vi "THzTimeScan_830_VC_PSD_TA_170401.vi"(0 "input":T1={"Step Number"=0, "Step"=0.0, "Start Position"=0.0, "Time-out"=0, "Lockin Address"="", "Short term \nAverage#"=0, "ESP300 Axis"=0, "error in"={"status"=FALSE, "code"=0, "source"=""}, "Value"="", "Delay"=0.0, "Delay2"=0.0, "savepath"=path "", "Power meter"={"ConexPSD Reference"=refnum, "error out"={"status"=FALSE, "code"=0, "source"=""}, "Component ID"=1}}) -> (1 "loop stop":bool, 2 "x-axis":sgl[](array[numeric]), 3 "y-axis":dbl[](array[numeric]), 4 "ext. out":cluster{dbl[], dbl[], dbl[], dbl[], string[]})   [LabVIEW 2010]
uses:
  C:/Users/NBTP/Desktop/Tai Anh/1. Courses + Small Works/Graduation Project/LabVIEW/TDS LabVIEW/THz Time(ESP300&SR830&PSD&MCS) TA_170209/Dll/Newport.CONEXPSD.CommandInterface.DLL
  THz Time(ESP300&SR830&PSD&MCS) TA_170209/Dll/Newport.CONEXPSD.CommandInterface.DLL
  <vilib>/Utility/file.llb/Write To Spreadsheet File (string).vi
panel:
  out "Power":dbl(graph)
  out "Y position":dbl(graph)
  out "X position":dbl(graph)
  out "Y pos.":dbl
  out "X pos.":dbl
  out "Pow.":dbl
  out "Position":dbl[](array[numeric])=[3.9963] format="%.6f"
  out "Array":dbl[](array[numeric])
  out "String":string
  out "Move delay":bool
  out "Read830":bool
  out "THz Signal Graph":dbl(graph)
  in  "loop stop":bool
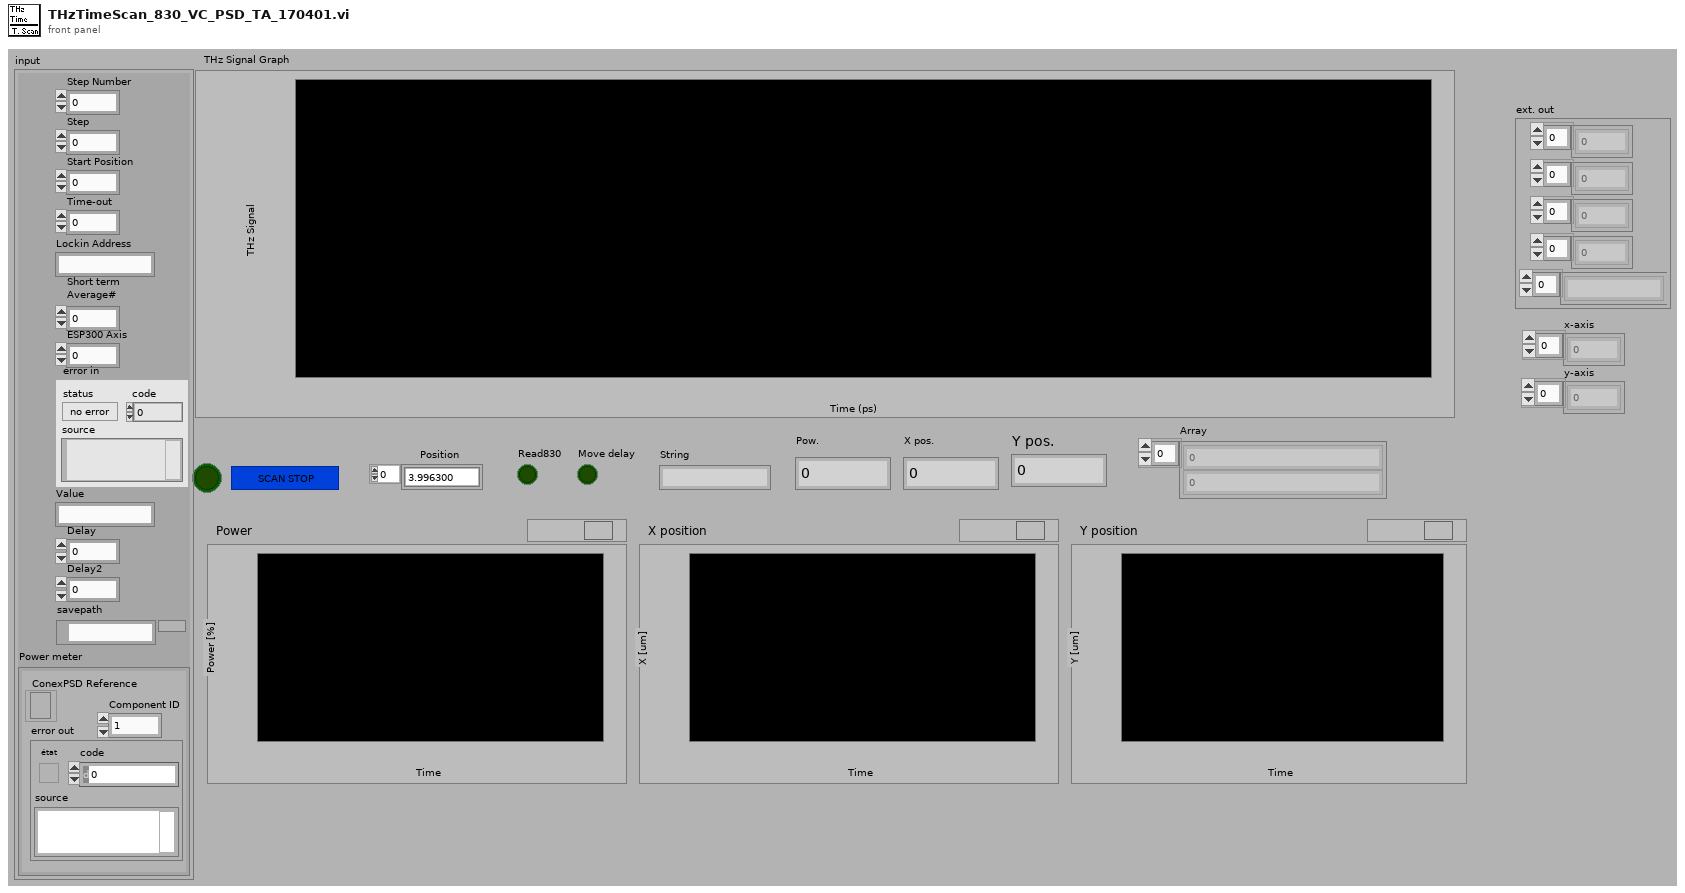
[diagram p1: front panel]
types:
  T1 = cluster{"Step Number":i32, "Step":sgl, "Start Position":sgl, "Time-out":i32, "Lockin Address":string, "Short term \nAverage#":i8, "ESP300 Axis":i8, "error in":errorcluster, "Value":string, "Delay":dbl, "Delay2":dbl, "savepath":path, "Power meter":cluster{"ConexPSD Reference":refnum<k24>, "error out":errorcluster, "Component ID":i32}}
  T2 = cluster{"ConexPSD Reference":refnum<k24>, "error out":errorcluster, "Component ID":i32}
  T3 = cluster{"PositionX":dbl, "PositionY":dbl, "LaserPower":dbl}
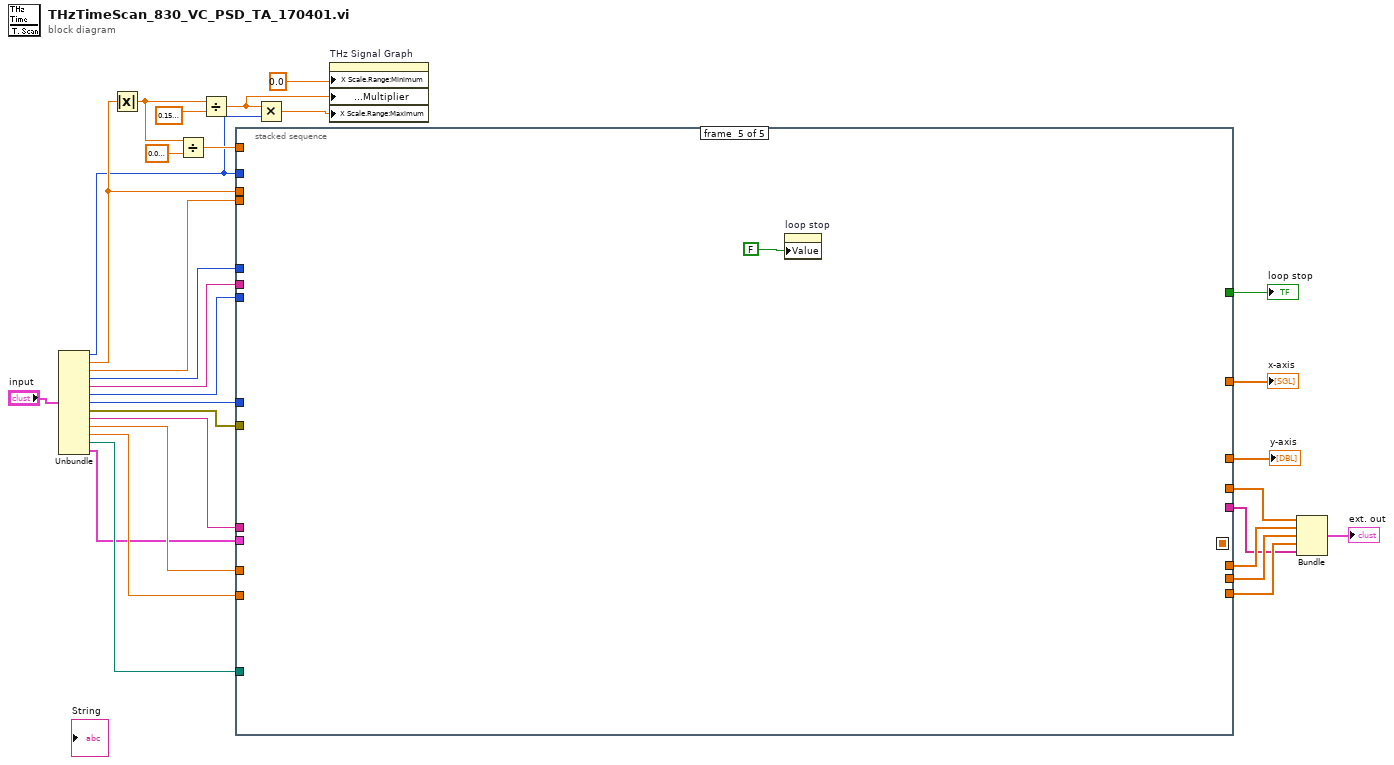
[diagram p0: block diagram]
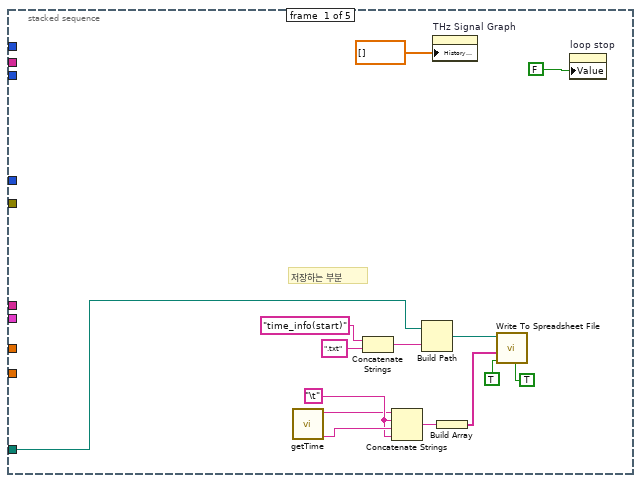
[diagram p2: hidden frame]
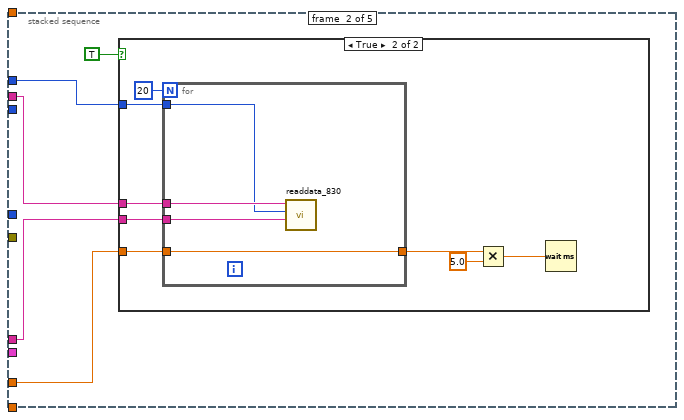
[diagram p3: hidden frame]
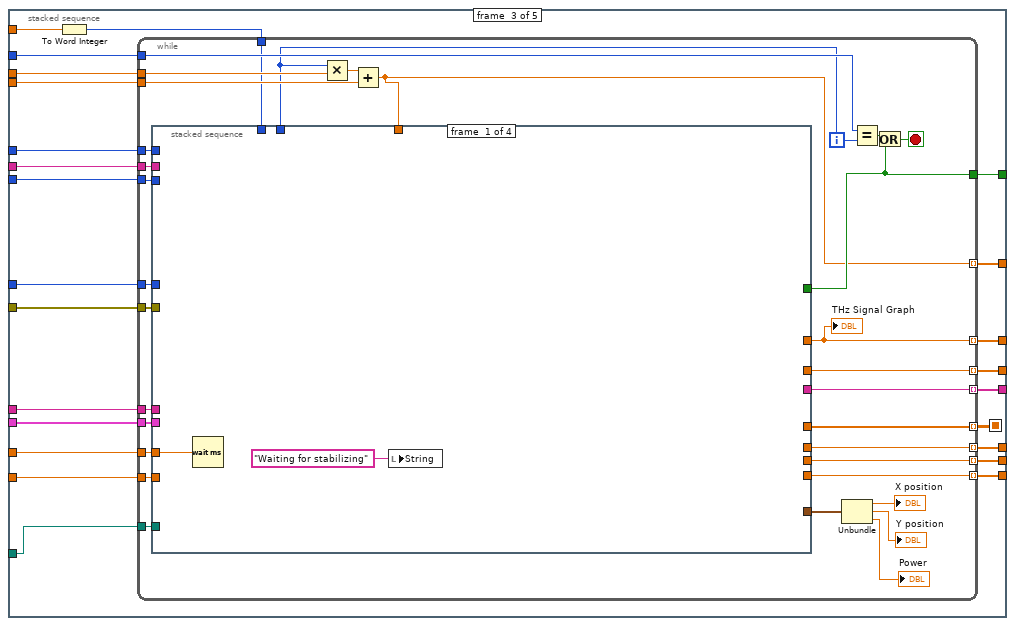
[diagram p5: hidden frame]
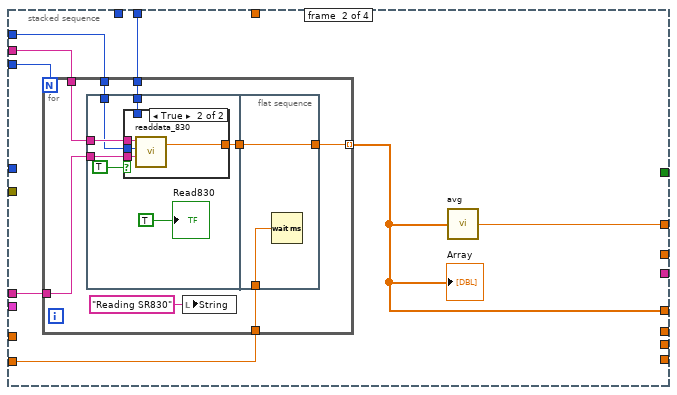
[diagram p6: hidden frame]
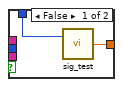
[diagram p7: hidden frame]
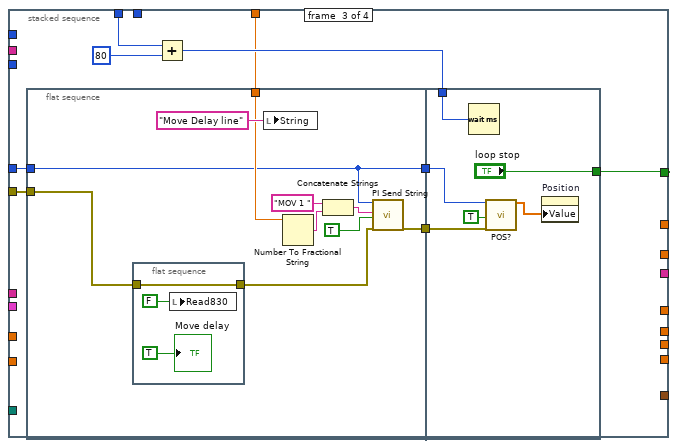
[diagram p8: hidden frame]
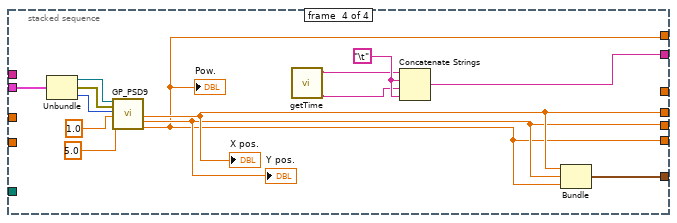
[diagram p9: hidden frame]
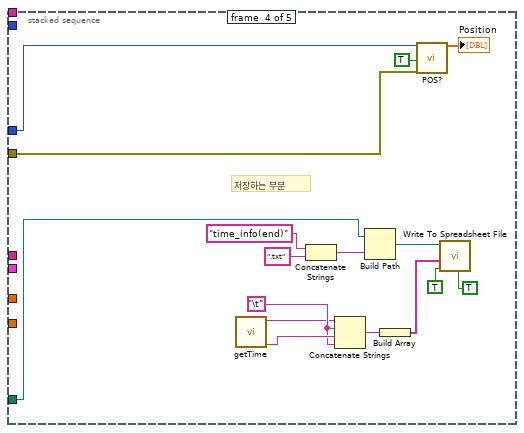
[diagram p10: hidden frame]
diagram:
  n1 = Unbundle("input") -> ("Step Number"=w16:i32, "Step"=w22:sgl, "Start Position"=w21:sgl, "Time-out"=w20:i32, "Lockin Address"=w19:string, "Short term \nAverage#"=w12:i8, "ESP300 Axis"=w18:i8, "error in"=w8:errorcluster, "Value"=w17:string, "Delay"=w11:dbl, "Delay2"=w10:dbl, "savepath"=w9:path, "Power meter"=w7:T2)
  n2 = Absolute Value(x=w22) -> (abs(x)=w26:sgl)
  n3 = Divide(x=w26, y=sgl 0.004) -> (x/y=w24:sgl)
  n4 = Divide(x=w26, y=sgl 0.15) -> (x/y=w14:sgl)
  n5 = stacked-sequence {
    seq-local: [_ _ w71 _ _] -> [_ _ _ _ _]
    tunnel: w21 -> [_ _ w85 _ _]
    tunnel: w20 -> [_ w49 w84 _ _]
    tunnel: w19 -> [_ w48 w83 _ _]
    tunnel: w12 -> [_ _ w82 _ _]
    tunnel: w18 -> [_ _ w69 w193 _]
    tunnel: w8 -> [_ _ w68 w192 _]
    tunnel: w17 -> [_ w47 w74 _ _]
    tunnel: [_ _ w81 _ _] -> w30
    tunnel: [_ _ w80 _ _] -> w29
    tunnel: [_ _ w79 _ _] -> w28
    tunnel: w22 -> [_ _ w77 _ _]
    tunnel: w16 -> [_ _ w78 _ _]
    tunnel: w24 -> [_ _ w76 _ _]
    tunnel: w11 -> [_ w45 w73 _ _]
    tunnel: w10 -> [_ _ w72 _ _]
    tunnel: w9 -> [w31 _ w70 w196 _]
    tunnel: w7 -> [_ _ w67 _ _]
    tunnel: [_ _ w66 _ _] -> w5
    tunnel: [_ _ w65 _ _] -> w4
    tunnel: [_ _ w64 _ _] -> w3
    tunnel: [_ _ w63 _ _] -> w2
    tunnel: [_ _ w62 _ _] -> w6
    frame #0 {
      w34 = "\t"
      # "저장하는 부분"
      n6 = call "getTime.vi"() -> ("시간"=w35:string, "날짜"=w33:string)  [unwired: 10 in]
      n7 = Concatenate Strings("time_info(start)" ("string"), ".txt" ("string")) -> (w41:string)
      n8 = Concatenate Strings(w33, w34, w35, w34) -> (w32:string)
      n9 = Build Path(base path=w31, name or relative path=w41) -> (appended path=w38:path)
      n10 = property on="THz Signal Graph" class="WFChart (strict)"("History Data"=dbl[] []) -> ()  [unwired: 2 in, 2 out]
      n11 = Build Array(w32) -> (w37:string[])
      n12 = call-poly <vilib>:"Write To Spreadsheet File.vi"("transpose? (no:F)"=TRUE ("transpose?\n(no:F)"), "append to file? (new file:F)"=TRUE ("transpose?\n(no:F)"), "1D data"=w37, "file path (dialog if empty)"=w38) -> ()  [unwired: 4 in, 1 out]
      n13 = property on="loop stop" class="Bool (strict)"("Value"=FALSE) -> ()  [unwired: 2 in, 2 out]
    }
    frame #1 {
      n14 = case shown="True" TRUE {
        tunnel: w49 -> [_ w56]
        tunnel: w48 -> [_ w55]
        tunnel: w47 -> [_ w54]
        tunnel: w45 -> [_ w53]
        frame False {
        }
        frame True {
          n15 = for {
            N: 20 -> [_]
            tunnel: w55 -> [w61]
            tunnel: w54 -> [w60]
            tunnel: w56 -> [w59]
            tunnel: w53 -> [w58]
            tunnel: [w58] -> w52
            n16 = call "readdata_830.vi"("Command"=w60, "timeout"=w59, "Lockin Address"=w61) -> ()  [unwired: 1 in, 2 out]
          }
          n17 = Multiply(x=w52, y=5.0) -> (x*y=w50:dbl)
          n18 = Wait (ms)(milliseconds to wait=w50) -> ()  [unwired: 1 out]
        }
      }
    }
    frame #2 {
      n19 = To Word Integer(number=w76) -> (16bit integer=w75:i16)
      n20 = while {
        tunnel: [w104] -> w81
        tunnel: [w108] -> w79 mode=indexing
        tunnel: [w98] -> w80 mode=indexing
        tunnel: w78 -> [w113]
        tunnel: w77 -> [w112]
        tunnel: w85 -> [w111]
        tunnel: w84 -> [w105]
        tunnel: w83 -> [w110]
        tunnel: w82 -> [w109]
        tunnel: w75 -> [w107]
        tunnel: w74 -> [w106]
        tunnel: w73 -> [w103]
        tunnel: w72 -> [w102]
        tunnel: [w101] -> w71 mode=indexing
        tunnel: w70 -> [w99]
        tunnel: w69 -> [w97]
        tunnel: w68 -> [w96]
        tunnel: w67 -> [w95]
        tunnel: [w90] -> w66 mode=indexing
        tunnel: [w89] -> w65 mode=indexing
        tunnel: [w88] -> w64 mode=indexing
        tunnel: [w87] -> w63 mode=indexing
        tunnel: [w86] -> w62 mode=indexing
        i -> [w100]
        stop <- w116 stop-if-true
        n21 = Multiply(x=w100, y=w112) -> (x*y=w114:sgl)
        n22 = Add(x=w114, y=w111) -> (x+y=w98:sgl)
        n23 = stacked-sequence {
          tunnel: w110 -> [_ w123 _ _]
          tunnel: [_ w125 _ _] -> w108
          tunnel: w109 -> [_ w126 _ _]
          tunnel: w107 -> [_ _ w158 _]
          tunnel: w106 -> [_ w124 _ _]
          tunnel: w105 -> [_ w122 _ _]
          tunnel: [_ _ w155 _] -> w104
          tunnel: w103 -> [w118 _ _ _]
          tunnel: w102 -> [_ w121 _ _]
          tunnel: [_ w120 _ _] -> w101
          tunnel: w100 -> [_ w119 _ _]
          tunnel: w99 -> [_ _ _ _]
          tunnel: w98 -> [_ _ w154 _]
          tunnel: w97 -> [_ _ w153 _]
          tunnel: w96 -> [_ _ w152 _]
          tunnel: w95 -> [_ _ _ w183]
          tunnel: [_ _ _ w179] -> w86
          tunnel: [_ _ _ w182] -> w87
          tunnel: [_ _ _ w181] -> w90
          tunnel: [_ _ _ w180] -> w89
          tunnel: [_ _ _ w179] -> w88
          tunnel: [_ _ _ w178] -> w91
          frame #0 {
            n24 = Wait (ms)(milliseconds to wait=w118) -> ()  [unwired: 1 out]
            n25 = local write "String"("Waiting for stabilizing" ("String")) -> ()
          }
          frame #1 {
            n26 = for {
              N: w126 -> [_]
              tunnel: w123 -> [w131]
              tunnel: w122 -> [w134]
              tunnel: [w133] -> w120 mode=indexing
              tunnel: w124 -> [w132]
              tunnel: w121 -> [w128]
              tunnel: w119 -> [w127]
              n27 = flat-sequence {
                tunnel: w134 -> [w138]
                tunnel: w132 -> [w139]
                tunnel: w131 -> [w140]
                tunnel: [w137] -> w129
                tunnel: w127 -> [w135]
                tunnel: [w149] -> w133
                tunnel: w129 -> [w149]
                tunnel: w128 -> [w148]
                frame #0 {
                  n28 = case shown="True" TRUE {
                    tunnel: w140 -> [_ w147]
                    tunnel: w139 -> [_ w146]
                    tunnel: w138 -> [_ w145]
                    tunnel: [w143 w144] -> w137
                    tunnel: w135 -> [w142 _]
                    frame False {
                      n29 = call "sig_test.vi"("index (row)"=w142) -> ("element"=w143:dbl)  [unwired: 1 in]
                    }
                    frame True {
                      n30 = call "readdata_830.vi"("Command"=w146, "timeout"=w145, "Lockin Address"=w147) -> ("Data"=w144:dbl)  [unwired: 1 in, 1 out]
                    }
                  }
                  "Read830" <- TRUE ("Read830")
                }
                frame #1 {
                  n31 = Wait (ms)(milliseconds to wait=w148) -> ()  [unwired: 1 out]
                }
              }
              n32 = local write "String"("Reading SR830" ("String")) -> ()
            }
            "Array" <- w120
            n33 = call "avg.vi"("Array"=w120) -> ("Numeric"=w125:dbl)
          }
          frame #2 {
            n34 = flat-sequence {
              tunnel: w154 -> [w163]
              tunnel: w153 -> [w159]
              tunnel: w152 -> [w162]
              tunnel: [w160] -> w151
              tunnel: [w159] -> w150
              tunnel: w157 -> [w176]
              tunnel: ["loop stop"] -> w155
              tunnel: w151 -> [w174]
              tunnel: w150 -> [w173]
              frame #0 {
                n35 = flat-sequence {
                  tunnel: [w171] -> w161
                  tunnel: w162 -> [w171]
                  frame #0 {
                    n36 = local write "Read830"(FALSE ("Read830")) -> ()
                    "Move delay" <- TRUE ("Move delay")
                  }
                }
                n37 = local write "String"("Move Delay line" ("String")) -> ()
                n38 = Number To Fractional String(number=w163) -> (F-format string=w167:string)  [unwired: 3 in]
                n39 = Concatenate Strings("MOV 1 ", w167) -> (w164:string)
                n40 = call "PI Send String.vi"("System no."=w159, "String to send"=w164, "Attach termination char.?"=TRUE ("Attach Linefeed?"), "error in"=w161) -> ("error out"=w160:errorcluster)  [unwired: 15 in]
              }
              frame #1 {
                n41 = Wait (ms)(milliseconds to wait=w176) -> ()  [unwired: 1 out]
                n42 = call "POS?.vi"("System no."=w173, "All axes?"=TRUE, "error in"=w174) -> ("Position"=w172:dbl[])  [unwired: 15 in, 1 out]
                n43 = property on="Position" class="Arr (strict)"("Value"=w172) -> ()  [unwired: 2 in, 2 out]
              }
            }
            n44 = Add(x=w158, y=i16 80) -> (x+y=w157:i16)
          }
          frame #3 {
            w186 = "\t"
            n45 = Unbundle(w183) -> ("ConexPSD Reference"=w191:refnum<k24>, "error out"=w190:errorcluster, "Component ID"=w189:i32)
            n46 = call "GP_PSD9.vi"("ConexPSD Reference"=w191, "error out"=w190, "Component ID"=w189, "Adress"=1.0, "shot average"=5.0) -> ("PositionX"=w181:dbl, "PositionY"=w180:dbl, "LaserPower"=w179:dbl)  [unwired: 8 in, 4 out]
            "Pow." <- w179
            "X pos." <- w181
            "Y pos." <- w180
            n47 = call "getTime.vi"() -> ("시간"=w184:string, "날짜"=w185:string)  [unwired: 10 in]
            n48 = Concatenate Strings(w185, w186, w184, w186) -> (w182:string)
            n49 = Bundle("PositionX"=w181, "PositionY"=w180, "LaserPower"=w179) -> (w178:T3)  [unwired: 1 in]
          }
        }
        "THz Signal Graph" <- w108
        n50 = Unbundle(w91) -> ("PositionX"=→"X position":dbl, "PositionY"=→"Y position":dbl, "LaserPower"=→"Power":dbl)
        n51 = Equal?(x=w113, y=w100) -> (x = y?=w115:bool)
        n52 = Or(x=w115, y=w104) -> (x .or. y?=w116:bool)
      }
    }
    frame #3 {
      w199 = "\t"
      # "저장하는 부분"
      n53 = call "getTime.vi"() -> ("시간"=w200:string, "날짜"=w198:string)  [unwired: 10 in]
      n54 = Concatenate Strings("time_info(end)" ("string"), ".txt" ("string")) -> (w206:string)
      n55 = Concatenate Strings(w198, w199, w200, w199) -> (w197:string)
      n56 = Build Path(base path=w196, name or relative path=w206) -> (appended path=w203:path)
      n57 = Build Array(w197) -> (w202:string[])
      n58 = call "POS?.vi"("System no."=w193, "All axes?"=TRUE, "error in"=w192) -> ("Position"=→"Position":dbl[])  [unwired: 15 in, 1 out]
      n59 = call-poly <vilib>:"Write To Spreadsheet File.vi"("transpose? (no:F)"=TRUE ("transpose?\n(no:F)"), "append to file? (new file:F)"=TRUE ("transpose?\n(no:F)"), "1D data"=w202, "file path (dialog if empty)"=w203) -> ()  [unwired: 4 in, 1 out]
    }
    frame #4 {
      n60 = property on="loop stop" class="Bool (strict)"("Value"=FALSE) -> ()  [unwired: 2 in, 2 out]
    }
  }
  "loop stop" <- w30
  "x-axis" <- w29
  "y-axis" <- w28
  n61 = Multiply(x=w14, y=w16) -> (x*y=w13:sgl)
  n62 = property on="THz Signal Graph" class="WFChart (strict)"("X Scale.Range:Minimum"=0.0, "X Scale.Offset and Multiplier:Multiplier"=w14, "X Scale.Range:Maximum"=w13) -> ()  [unwired: 2 in, 2 out]
  n63 = Bundle(w6, w5, w4, w3, w2) -> (→"ext. out":cluster{dbl[], dbl[], dbl[], dbl[], string[]})  [unwired: 1 in]
